vi "Write Last Waveforms.vi"(8 "error in (no error)":errorcluster, 10 "Last Waveforms":map{u8, waveform(dbl)}(c390), 11 "Thermometer DAQmx in":refnum<class "Thermometer DAQmx.lvclass">) -> (0 "error out":errorcluster, 3 "Thermometer DAQmx out":refnum<class "Thermometer DAQmx.lvclass">)   [LabVIEW 2023, in "Thermometer.lvlib" / "Thermometer DAQmx.lvlib" / "Thermometer DAQmx.lvclass"]
uses:
  Thermometer DAQmx.lvclass
  Thermometer DAQmx.lvclass/Thermometer DAQmx.ctl
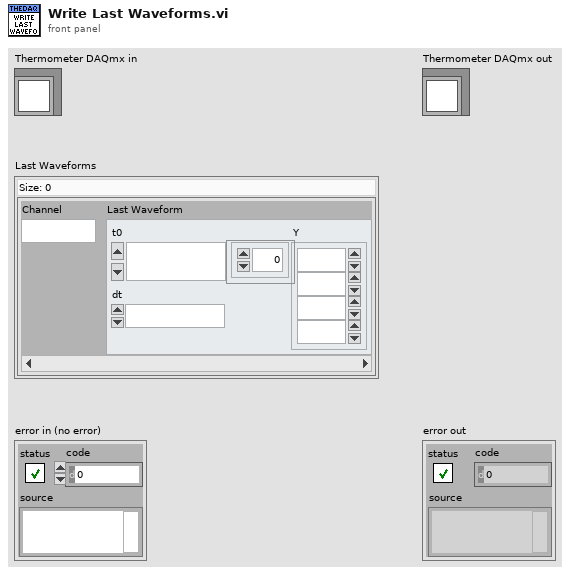
[diagram p1: front panel]
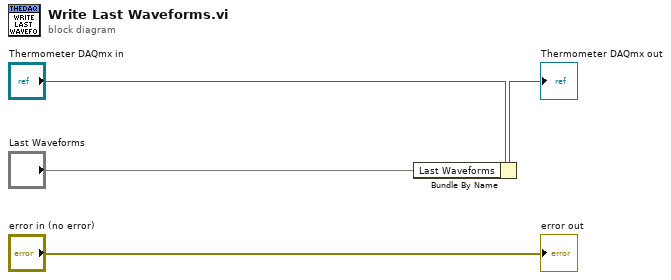
[diagram p0: block diagram]
diagram:
  n1 = Bundle By Name(cluster="Thermometer DAQmx in", "Last Waveforms"="Last Waveforms") -> (→"Thermometer DAQmx out":refnum<class "Thermometer DAQmx.lvclass">)
  "error out" <- "error in (no error)"
